vi "SBG_Ellipse_skip_data_if_incorrect (SubVI).vi"(2 "String":string, 4 "result string in":string) -> (0 "Data skipped":bool, 1 "result string out":string)   [LabVIEW 2017]
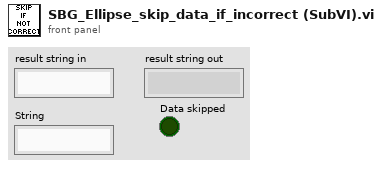
[diagram p1: front panel]
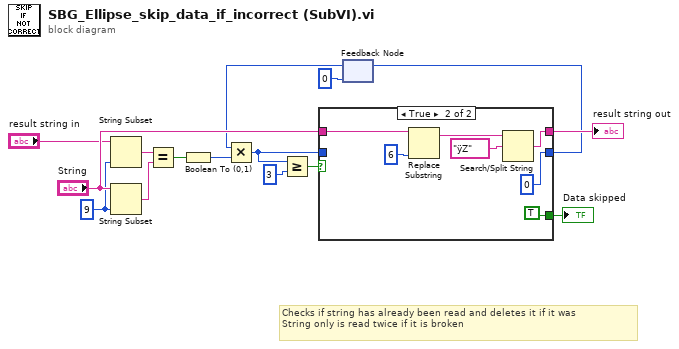
[diagram p0: block diagram]
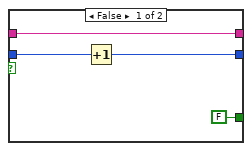
[diagram p2: hidden frame]
diagram:
  w12 = 9 ("length (rest)")
  # "Checks if string has already been read and deletes it if it was\nString only is read twice if it is broken"
  n1 = String Subset(string="result string in", length (rest)=w12) -> (substring=w14:string)  [unwired: 1 in]
  n2 = String Subset(string="String", length (rest)=w12) -> (substring=w13:string)  [unwired: 1 in]
  n3 = Equal?(x=w14, y=w13) -> (x = y?=w9:bool)
  n4 = Boolean To (0,1)(Boolean=w9) -> (0, 1=w8:i16)
  n5 = feedback #1(i16 0) -> (w7:i16)
  n6 = Multiply(x=w7, y=w8) -> (x*y=w4:i16)
  n7 = Greater Or Equal?(x=w4, y=i16 3) -> (x >= y?=w2:bool)
  n8 = case shown="True" w2 {
    tunnel: "String" -> [w19 w26]
    tunnel: [w19 w23] -> w10
    tunnel: [w17 i16 0] -> w6
    tunnel: w4 -> [w18 _]
    tunnel: [FALSE TRUE] -> w1
    frame False {
      n9 = Increment(x=w18) -> (x+1=w17:i16)
    }
    frame True {
      n10 = Replace Substring(2:6 ("length (len. of substring)"), 5:w26) -> (1:w24:string)  [unwired: 2 in, 1 out]
      n11 = Search/Split String(string=w24, search string/char (-)="ÿZ") -> (match + rest of string=w23:string)  [unwired: 1 in, 2 out]
    }
  }
  "result string out" <- w10
  "Data skipped" <- w1
  n12 = feedback-in #1(w6) -> ()
